vi "test-quintic-spline-03b.vi"() -> (3 "Test Passed":bool)   [LabVIEW 2019]
uses:
  <vilib>/Rock Robotics/WPI/ThirdParty/JAS_Junk/TrajLib/POSEwCURVATURE.ctl
  <vilib>/Rock Robotics/WPI/ThirdParty/JAS_Junk/TrajLib/POSE2D.ctl
  <vilib>/Rock Robotics/WPI/ThirdParty/JAS_Junk/TrajLib/TRANSLATION2D.ctl
  <vilib>/Rock Robotics/WPI/ThirdParty/JAS_Junk/TrajLib/ROTATION2D.ctl
  <vilib>/Rock Robotics/WPI/ThirdParty/JAS_Junk/TrajLib/Rotation2d_CreateAngle.vi
  <vilib>/Rock Robotics/WPI/ThirdParty/JAS_Junk/TrajLib/Translation2d_Create.vi
  <vilib>/Rock Robotics/WPI/ThirdParty/JAS_Junk/TrajLib/Util_CalcDist.vi
  <vilib>/Rock Robotics/WPI/ThirdParty/JAS_Junk/TrajLib/Trajectory_Library.lvlib
panel:
  out "XY Graph":cluster{dbl[], dbl[]}(graph)
  out "Numb\nWaypoints":i32
  out "All Interior \nwayPoints\nFound (True)":bool
  out "end rot = 0":dbl
  out "end y = 0":dbl
  out "end x = 0":dbl
  out "start rot = 0":dbl
  out "start y = 0":dbl
  out "start x = 0":dbl
  out "max dtheta < 0.0872":dbl
  out "max dy < 0.00127":dbl
  out "max dx  < 0.127":dbl
  out "Overall Error":errorcluster
  out "Elements":i32
  out "Create Spline Error":errorcluster
  out "SplinePoses\nWCurve":T1[](array[typedef]) {"POSE"."ROTATION"."SIN" format="%13.4f"; "POSE"."ROTATION"."COS" format="%13.4f"; "POSE"."ROTATION"."VALUE" format="%13.4f"; "POSE"."TRANSLATION"."Y" format="%14.3f"; "POSE"."TRANSLATION"."X" format="%14.3f"}
  out "Elapsed Time":dbl
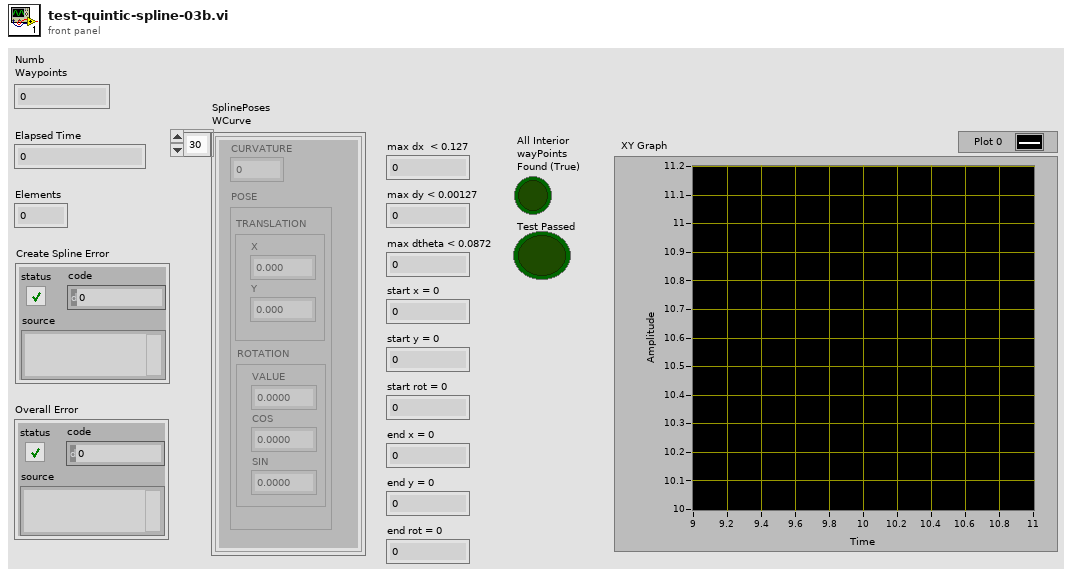
[diagram p1: front panel]
types:
  T1 = typedef "Trajectory_Library.lvlib/POSEwCURVATURE.ctl" = cluster{"CURVATURE":dbl, "POSE":T2}
  T2 = typedef "Trajectory_Library.lvlib/POSE2D.ctl" = cluster{"TRANSLATION":T3, "ROTATION":T4}
  T3 = typedef "Trajectory_Library.lvlib/TRANSLATION2D.ctl" = cluster{"X":dbl, "Y":dbl}
  T4 = typedef "Trajectory_Library.lvlib/ROTATION2D.ctl" = cluster{"VALUE":dbl, "COS":dbl, "SIN":dbl}
  T5 = typedef "Trajectory_Library.lvlib/SPLINE.ctl" = cluster{"Degree":i32, "Coefficients":T6}
  T6 = typedef "NI_Matrix.lvlib/RealMatrix.ctl" = dbl[][]
  T7 = typedef "Trajectory_Library.lvlib/TWIST2D.ctl" = cluster{"dX":dbl, "dY":dbl, "dTHETA":dbl}
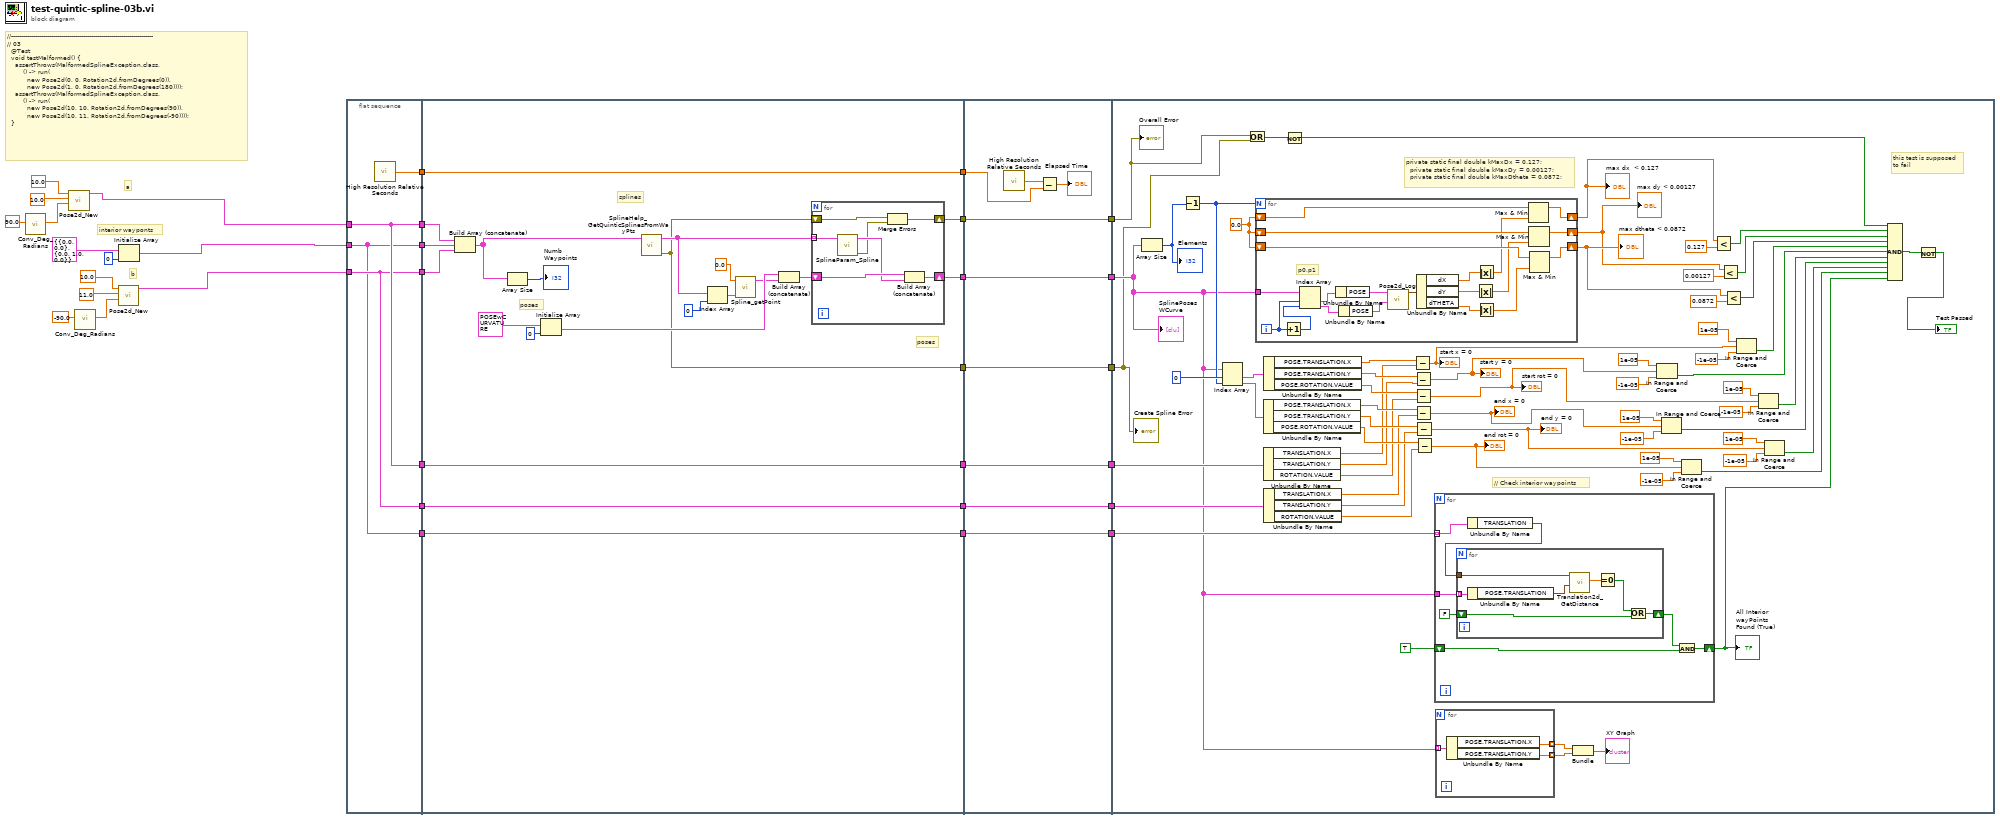
[diagram p0: block diagram]
diagram:
  # "interior wayponts"
  # "b"
  # "a"
  # "//-----------------------------------------------------------------------\n// 03\n  @Test\n  void testMalformed() {\n    assertThrows(MalformedSplineException.class,\n        () -> run(\n          new Pose2d(0, 0, Rotation2d.fromDegrees(0)),\n          new Pose2d(1, 0, Rotation2d.fromDegrees(180))));\n    assertThrows(MalformedSplineException.class,\n        () -> run(\n          new Pose2d(10, 10, Rotation2d.fromDegrees(90)),\n          new Pose2d(10, 11, Rotation2d.fromDegrees(-90))));\n  }"
  n1 = call <vilib>:"Conv_Deg_Radians.vi"("Degress"=90.0) -> ("Radians"=w6:dbl)  [unwired: 10 in]
  n2 = call <vilib>:"Pose2d_New.vi"("Heading"=w6, "Y"=10.0, "X"=10.0) -> ("out POSe"=w1:T2)  [unwired: 8 in]
  n3 = call <vilib>:"Conv_Deg_Radians.vi"("Degress"=-90.0) -> ("Radians"=w9:dbl)  [unwired: 10 in]
  n4 = call <vilib>:"Pose2d_New.vi"("Heading"=w9, "Y"=11.0, "X"=10.0) -> ("out POSe"=w3:T2)  [unwired: 8 in]
  n5 = Initialize Array(T2 {"TRANSLATION"={"X"=0.0, "Y"=0.0}, "ROTATION"={"VALUE"=0.0, "COS"=1.0, "SIN"=0.0}} ("POSE"), 0 ("dimension size")) -> (w2:T2[])
  n6 = flat-sequence {
    tunnel: w1 -> [w36]
    tunnel: [w36] -> w33
    tunnel: w3 -> [w35]
    tunnel: [w35] -> w32
    tunnel: [w37] -> w31
    tunnel: [w36] -> w23
    tunnel: [w35] -> w20
    tunnel: [w34] -> w15
    tunnel: w2 -> [w34]
    tunnel: [w34] -> w14
    tunnel: w33 -> [w42]
    tunnel: w32 -> [w41]
    tunnel: [w58] -> w30
    tunnel: w31 -> [w58]
    tunnel: [w48] -> w29
    tunnel: [w47] -> w27
    tunnel: [w46] -> w25
    tunnel: w23 -> [w45]
    tunnel: [w45] -> w22
    tunnel: w20 -> [w44]
    tunnel: [w44] -> w19
    tunnel: [w43] -> w16
    tunnel: w15 -> [w43]
    tunnel: w14 -> [w39]
    tunnel: w30 -> [w74]
    tunnel: w29 -> [w73]
    tunnel: [w73] -> w28
    tunnel: w27 -> [w72]
    tunnel: [w72] -> w26
    tunnel: w25 -> [w71]
    tunnel: [w71] -> w24
    tunnel: w22 -> [w68]
    tunnel: [w68] -> w21
    tunnel: w19 -> [w67]
    tunnel: [w67] -> w18
    tunnel: [w66] -> w17
    tunnel: w16 -> [w66]
    tunnel: w28 -> [w116]
    tunnel: w26 -> [w104]
    tunnel: w24 -> [w103]
    tunnel: w21 -> [w138]
    tunnel: w18 -> [w137]
    tunnel: w17 -> [w120]
    frame #0 {
      n7 = call <vilib>:"High Resolution Relative Seconds.vi"() -> ("relative seconds"=w37:dbl)
    }
    frame #1 {
      # "poses"
      # "poses"
      # "splines"
      n8 = Build Array (concatenate)(w42, w39, w41) -> (w38:T2[])
      n9 = Array Size(array=w38) -> (size(s)=→"Numb\nWaypoints":i32)
      n10 = Initialize Array(T1 {"CURVATURE"=0.0, "POSE"={"TRANSLATION"={"X"=0.0, "Y"=0.0}, "ROTATION"={"VALUE"=0.0, "COS"=1.0, "SIN"=0.0}}} ("POSEwCURVATURE"), 0 ("dimension size")) -> (w52:T1[])
      n11 = call <vilib>:"SplineHelp_GetQuinticSplinesFromWayPts.vi"("WayPoints"=w38) -> ("out Error"=w47:errorcluster, "Splines"=w49:T5[])  [unwired: 9 in]
      n12 = Index Array(array=w49, index=0) -> (element=w54:T5)
      n13 = call <vilib>:"Spline_getPoint.vi"("inputSPLINE"=w54, "Time"=0.0) -> ("POSEwCURVATURE"=w51:T1)  [unwired: 9 in]
      n14 = Build Array (concatenate)(w52, w51) -> (w50:T1[])
      n15 = for {
        shift-right: [w62] -> w48
        shift-left: w50 -> [w64]
        tunnel: w49 -> [w65] mode=indexing
        shift-right: [w60] -> w46
        shift-left: w47 -> [w61]
        n16 = call <vilib>:"SplineParam_Spline.vi"("inputSPLINE"=w65) -> ("error out"=w59:errorcluster, "outputPOSEwCURVATURE"=w63:T1[])  [unwired: 9 in]
        n17 = Merge Errors(w61, w59) -> (w60:errorcluster)
        n18 = Build Array (concatenate)(w64, w63) -> (w62:T1[])
      }
    }
    frame #2 {
      n19 = call <vilib>:"High Resolution Relative Seconds.vi"() -> ("relative seconds"=w69:dbl)
      n20 = Subtract(x=w69, y=w74) -> (x-y=→"Elapsed Time":dbl)
    }
    frame #3 {
      w139 = 0.0
      # "this test is supposed\nto fail"
      # "// Check interior waypoints"
      # "private static final double kMaxDx = 0.127;\n  private static final double kMaxDy = 0.00127;\n  private static final double kMaxDtheta = 0.0872;"
      n21 = Array Size(array=w116) -> (size(s)=w140:i32)
      "Elements" <- w140
      n22 = Decrement(x=w140) -> (x-1=w135:i32)
      n23 = Index Array(array=w116, index #1=0 ("index"), index #2=w135) -> (element #1=w134:T1, element #2=w133:T1)
      n24 = Or(x=w103, y=w104) -> (x .or. y?=w105:bool)
      n25 = for {
        N: w135 -> [_]
        tunnel: w116 -> [w175]
        shift-right: [w166] -> w109
        shift-left: w139 -> [w163]
        shift-right: [w164] -> w111
        shift-left: w139 -> [w161]
        shift-right: [w165] -> w110
        shift-left: w139 -> [w162]
        i -> [w177]
        # "p0,p1"
        n26 = Increment(x=w177) -> (x+1=w176:i32)
        n27 = Index Array(array=w175, index #1=w177, index #2=w176) -> (element #1=w174:T1, element #2=w173:T1)
        n28 = Unbundle By Name(w174) -> ("POSE"=w172:T2)
        n29 = Unbundle By Name(w173) -> ("POSE"=w171:T2)
        n30 = call <vilib>:"Pose2d_Log.vi"("end POSE"=w171, "in POSE"=w172) -> ("out TWIST"=w170:T7)  [unwired: 9 in]
        n31 = Unbundle By Name(w170) -> ("dX"=w167:dbl, "dY"=w168:dbl, "dTHETA"=w169:dbl)
        n32 = Absolute Value(x=w168) -> (abs(x)=w159:dbl)
        n33 = Absolute Value(x=w167) -> (abs(x)=w160:dbl)
        n34 = Absolute Value(x=w169) -> (abs(x)=w158:dbl)
        n35 = Max & Min(x=w163, y=w160) -> (max(x,y)=w166:dbl)  [unwired: 1 out]
        n36 = Max & Min(x=w162, y=w159) -> (max(x,y)=w165:dbl)  [unwired: 1 out]
        n37 = Max & Min(x=w161, y=w158) -> (max(x,y)=w164:dbl)  [unwired: 1 out]
      }
      "max dx  < 0.127" <- w109
      "max dy < 0.00127" <- w110
      "max dtheta < 0.0872" <- w111
      n38 = Unbundle By Name(w133) -> ("POSE.TRANSLATION.X"=w129:dbl, "POSE.TRANSLATION.Y"=w128:dbl, "POSE.ROTATION.VALUE"=w127:dbl)
      n39 = Unbundle By Name(w138) -> ("TRANSLATION.X"=w126:dbl, "TRANSLATION.Y"=w125:dbl, "ROTATION.VALUE"=w124:dbl)
      n40 = Unbundle By Name(w134) -> ("POSE.TRANSLATION.X"=w132:dbl, "POSE.TRANSLATION.Y"=w131:dbl, "POSE.ROTATION.VALUE"=w130:dbl)
      n41 = Unbundle By Name(w137) -> ("TRANSLATION.X"=w123:dbl, "TRANSLATION.Y"=w122:dbl, "ROTATION.VALUE"=w121:dbl)
      n42 = Not(x=w105) -> (.not. x?=w102:bool)
      n43 = Subtract(x=w132, y=w126) -> (x-y=w98:dbl)
      "start x = 0" <- w98
      n44 = Subtract(x=w131, y=w125) -> (x-y=w77:dbl)
      "start y = 0" <- w77
      n45 = Subtract(x=w130, y=w124) -> (x-y=w81:dbl)
      "start rot = 0" <- w81
      n46 = Subtract(x=w129, y=w123) -> (x-y=w82:dbl)
      "end x = 0" <- w82
      n47 = Subtract(x=w128, y=w122) -> (x-y=w89:dbl)
      "end y = 0" <- w89
      n48 = Subtract(x=w127, y=w121) -> (x-y=w93:dbl)
      "end rot = 0" <- w93
      n49 = for {
        tunnel: w120 -> [w145] mode=indexing
        tunnel: w116 -> [w150]
        shift-right: [w149] -> w101
        shift-left: TRUE -> [w148]
        n50 = Unbundle By Name(w145) -> ("TRANSLATION"=w144:T3)
        n51 = for {
          tunnel: w150 -> [w154] mode=indexing
          shift-right: [w157] -> w146
          shift-left: FALSE -> [w156]
          tunnel: w144 -> [w155]
          n52 = Unbundle By Name(w154) -> ("POSE.TRANSLATION"=w153:T3)
          n53 = call <vilib>:"Translation2d_GetDistance.vi"("other Translation"=w153, "In Translation"=w155) -> ("Distance"=w152:dbl)  [unwired: 9 in]
          n54 = Equal To 0?(x=w152) -> (x = 0?=w151:bool)
          n55 = Or(x=w151, y=w156) -> (x .or. y?=w157:bool)
        }
        n56 = And(x=w146, y=w148) -> (x .and. y?=w149:bool)
      }
      "All Interior \nwayPoints\nFound (True)" <- w101
      n57 = for {
        tunnel: [w143] -> w118 mode=indexing
        tunnel: [w142] -> w117 mode=indexing
        tunnel: w116 -> [w141] mode=indexing
        n58 = Unbundle By Name(w141) -> ("POSE.TRANSLATION.X"=w143:dbl, "POSE.TRANSLATION.Y"=w142:dbl)
      }
      n59 = Bundle(w118, w117) -> (→"XY Graph":cluster{dbl[], dbl[]})  [unwired: 1 in]
      n60 = In Range and Coerce(upper limit=1e-05, x=w77, lower limit=-1e-05) -> (In Range?=w78:bool)  [unwired: 1 out]
      n61 = In Range and Coerce(upper limit=1e-05, x=w82, lower limit=-1e-05) -> (In Range?=w84:bool)  [unwired: 1 out]
      n62 = In Range and Coerce(upper limit=1e-05, x=w93, lower limit=-1e-05) -> (In Range?=w94:bool)  [unwired: 1 out]
      n63 = Less?(x=w109, y=0.127) -> (x < y?=w108:bool)
      n64 = Less?(x=w110, y=0.00127) -> (x < y?=w107:bool)
      n65 = Less?(x=w111, y=0.0872) -> (x < y?=w106:bool)
      n66 = In Range and Coerce(upper limit=1e-05, x=w98, lower limit=-1e-05) -> (In Range?=w97:bool)  [unwired: 1 out]
      n67 = In Range and Coerce(upper limit=1e-05, x=w81, lower limit=-1e-05) -> (In Range?=w83:bool)  [unwired: 1 out]
      n68 = In Range and Coerce(upper limit=1e-05, x=w89, lower limit=-1e-05) -> (In Range?=w90:bool)  [unwired: 1 out]
      n69 = Compound Arithmetic op=AND(w102, w108, w107, w106, w97, w78, w83, w84, w90, w94, w101) -> (w76:bool)
      n70 = Not(x=w76) -> (.not. x?=→"Test Passed":bool)
      "SplinePoses\nWCurve" <- w116
      "Create Spline Error" <- w104
      "Overall Error" <- w103
    }
  }
